vi "Labview2020ExampleForOceanDirect.vi"() -> ()   [LabVIEW 2021]
uses:
  C:/Program Files/Ocean Insight/OceanDirect SDK/lib/NetOceanDirect.dll
  Program Files/Ocean Insight/OceanDirect SDK/lib/NetOceanDirect.dll
panel:
  in  "Integration time (us)":u32=10000
  in  "Use this stop button and not the LabVIEW abort button to allow clean up code to be exicuted":bool
  out "Spectrum":T1(graph)
  # "Simple demostration of using OceanDirect in LabVIEW via the .NET interface"
  # "See back panel for details on how to set up this deomonstration"
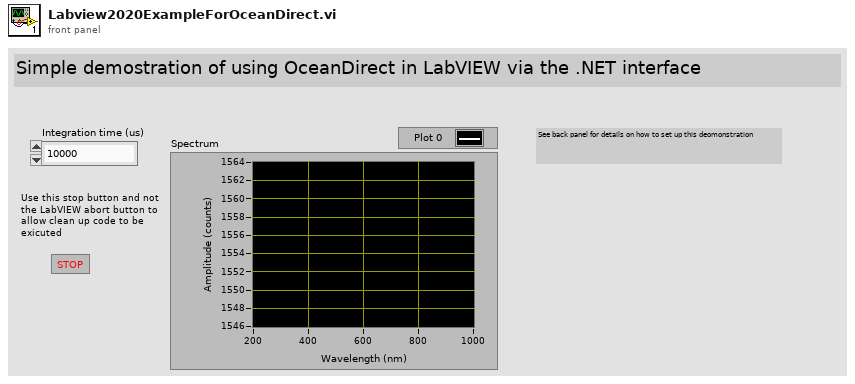
[diagram p1: front panel]
types:
  T1 = cluster{"getWavelengths":dbl[], "getSpectrum":dbl[]}
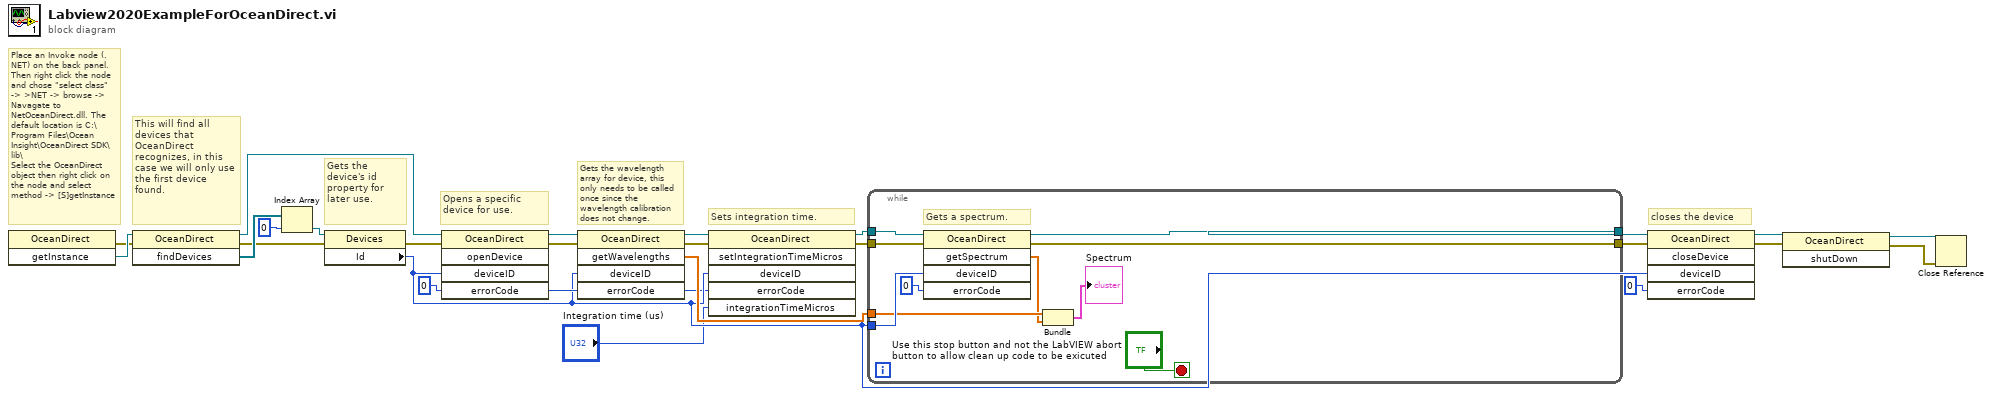
[diagram p0: block diagram]
diagram:
  # "closes the device"
  # "Place an Invoke node (.NET) on the back panel. Then right click the node and chose \"select class\" -> >NET -> browse -> Navagate to NetOceanDirect.dll. The default location is C:\\Program Files\\Ocean Insight\\OceanDirect SDK\\lib\\\nSelect the OceanDirect object then right click on the node and select method -> [S]getInstance"
  # "Sets integration time."
  # "Gets the wavelength array for device, this only needs to be called once since the wavelength calibration does not change."
  # "Opens a specific device for use."
  # "Gets the device's id property for later use."
  # "This will find all devices that OceanDirect recognizes, in this case we will only use the first device found."
  n1 = invoke class="OceanDirect" method="getInstance"() -> (error out=w14:errorcluster, "getInstance"=w15:refnum<k24>)  [unwired: 3 in, 1 out]
  n2 = invoke class="OceanDirect" method="findDevices"(reference=w15, error in=w14) -> (reference out=w21:refnum<k24>, error out=w19:errorcluster, "findDevices"=w27:refnum<k24>[])  [unwired: 1 in]
  n3 = Index Array(array=w27, index=0) -> (element=w25:refnum<k24>)
  n4 = property class="Devices"(reference=w25, error in=w19) -> (error out=w18:errorcluster, "Id"=w12:i32)  [unwired: 1 out]
  n5 = invoke class="OceanDirect" method="openDevice"(reference=w21, error in=w18, "deviceID"=w12, "errorCode"=0) -> (reference out=w16:refnum<k24>, error out=w7:errorcluster, "errorCode"=w17:i32)  [unwired: 1 in, 2 out]
  n6 = invoke class="OceanDirect" method="getWavelengths"(reference=w16, error in=w7, "deviceID"=w12, "errorCode"=w17) -> (reference out=w8:refnum<k24>, error out=w9:errorcluster, "getWavelengths"=w13:dbl[], "errorCode"=w11:i32)  [unwired: 1 in, 1 out]
  n7 = invoke class="OceanDirect" method="setIntegrationTimeMicros"(reference=w8, error in=w9, "deviceID"=w12, "errorCode"=w11, "integrationTimeMicros"="Integration time (us)") -> (reference out=w6:refnum<k24>, error out=w5:errorcluster)  [unwired: 1 in, 4 out]
  n8 = while {
    tunnel: [w36] -> w23
    tunnel: w12 -> [w35]
    tunnel: w13 -> [w31]
    tunnel: w6 -> [w34]
    tunnel: [w33] -> w20
    tunnel: w5 -> [w28]
    stop <- "Use this stop button and not the LabVIEW abort button to allow clean up code to be exicuted" stop-if-true
    # "Gets a spectrum."
    n9 = invoke class="OceanDirect" method="getSpectrum"(reference=w34, error in=w28, "deviceID"=w35, "errorCode"=0) -> (reference out=w33:refnum<k24>, error out=w36:errorcluster, "getSpectrum"=w30:dbl[])  [unwired: 1 in, 2 out]
    n10 = Bundle("getWavelengths"=w31, "getSpectrum"=w30) -> (→"Spectrum":T1)  [unwired: 1 in]
  }
  n11 = invoke class="OceanDirect" method="closeDevice"(reference=w20, error in=w23, "deviceID"=w12, "errorCode"=0) -> (reference out=w4:refnum<k24>, error out=w3:errorcluster)  [unwired: 1 in, 3 out]
  n12 = invoke class="OceanDirect" method="shutDown"(reference=w4, error in=w3) -> (reference out=w2:refnum<k24>, error out=w1:errorcluster)  [unwired: 1 in, 1 out]
  n13 = Close Reference(reference=w2, error in (no error)=w1) -> ()  [unwired: 1 out]
